vi "Implement Build Configuration.vi"(7 "Target in":refnum<vi>, 8 "error in (no error)":errorcluster, 10 "Build Config":T1, 11 "PPL in":refnum<class "NI_AB_API_PPL.lvclass">) -> (0 "error out":errorcluster, 3 "PPL out":refnum<class "NI_AB_API_PPL.lvclass">, 5 "Target out":refnum<vi>)   [LabVIEW 2019, in "PPL INI Parsing.lvlib"]
uses:
  PPL INI Parsing.lvlib
  Build Configuration.ctl
  <vilib>/AppBuilder/AB_API/PPL/NI_AB_API_PPL.lvclass
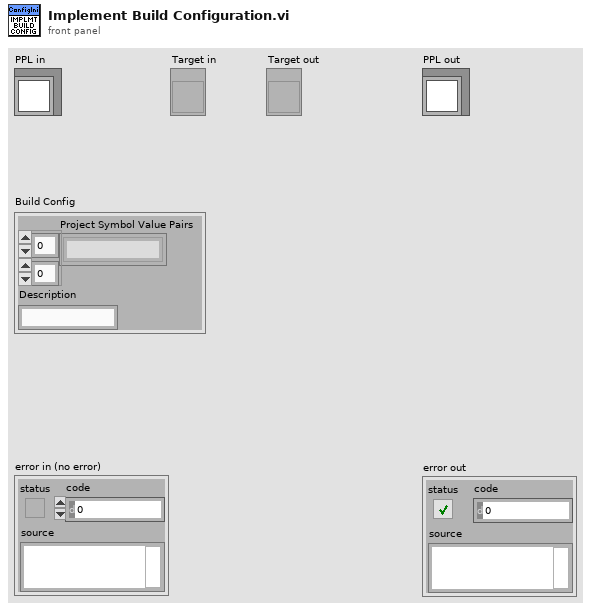
[diagram p1: front panel]
types:
  T1 = typedef "PPL INI Parsing.lvlib/Build Configuration.ctl" = cluster{"SV Pairs":string[][], "Description":string}
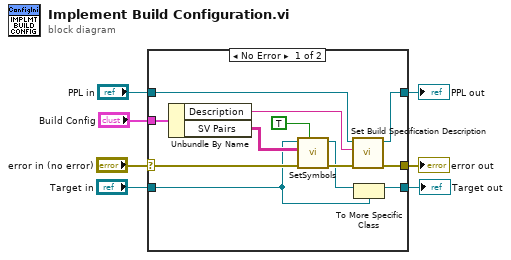
[diagram p0: block diagram]
diagram:
  n1 = case shown="No Error" "error in (no error)" {
    selector: "error in (no error)" -> [w10 w22]
    tunnel: "Build Config" -> [w19 _]
    tunnel: "PPL in" -> [w18 w21]
    tunnel: [w17 w21] -> w5
    tunnel: [w15 w22] -> w4
    tunnel: "Target in" -> [w8 w20]
    tunnel: [w9 w20] -> w2
    frame No Error {
      n2 = Unbundle By Name(w19) -> ("Description"=w16:string, "SV Pairs"=w11:string[][])
      n3 = call <resource>:"SetSymbols.vi"("Is Persistant? (FALSE)"=TRUE, "error in"=w10, "Symbol Value Pairs"=w11, "Project Item"=w8) -> ("error out"=w14:errorcluster, "Project Item"=w12:refnum<vi>)  [unwired: 6 in]
      n4 = call-dynamic "Set Build Specification Description.vi"("error in (no error)"=w14, "Build Specification Description"=w16, "NI_AB_API_PPL in"=w18) -> ("error out"=w15:errorcluster, "NI_AB_API_PPL out"=w17:refnum<class "NI_AB_API_PPL.lvclass">)  [unwired: 7 in]
      n5 = To More Specific Class(target class=w8, reference=w12) -> (specific class reference=w9:refnum<vi>)  [unwired: 1 in, 1 out]
    }
    frame Error {
    }
  }
  "error out" <- w4
  "Target out" <- w2
  "PPL out" <- w5
